vi "多帧发送机制(EV05).vi"(0 "can卡类型":u8, 1 "设备索引号":u8, 2 "CAN端口":u8, 3 "命令":u8 format="%x", 4 "板号":u8 format="%x", 5 "命令序号":u32, 6 "输入数据":dbl[](array[numeric]), 7 "错误输入（无错误）":errorcluster) -> (14 "错误代码":u32, 15 "总发送帧数":i32, 19 "错误输出":errorcluster)   [LabVIEW 2013]
uses:
  data/kerneldlls/usbcan.dll
panel:
  out "发送成功":bool
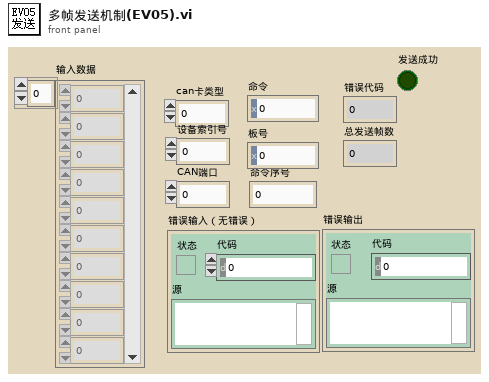
[diagram p1: front panel]
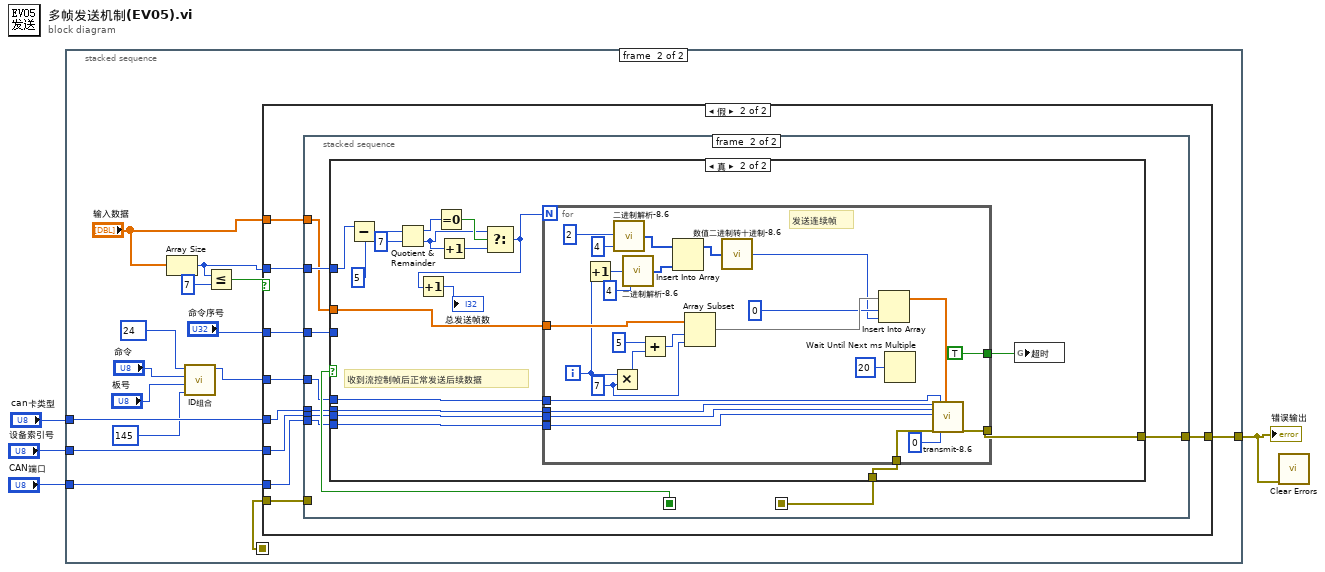
[diagram p0: block diagram]
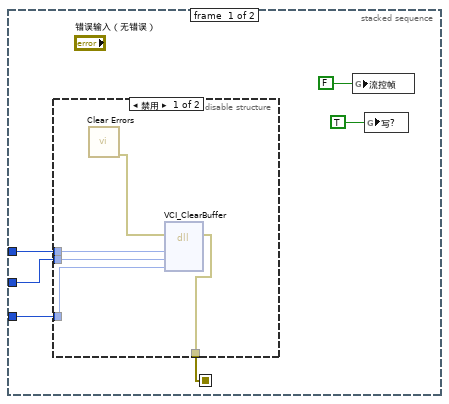
[diagram p2: hidden frame]
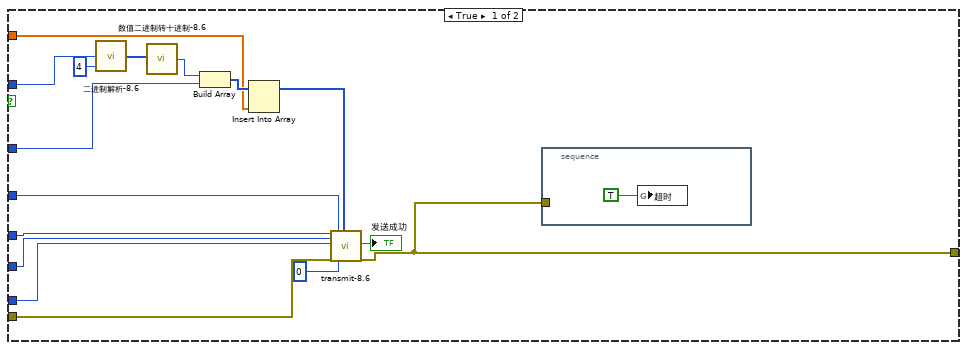
[diagram p4: hidden frame]
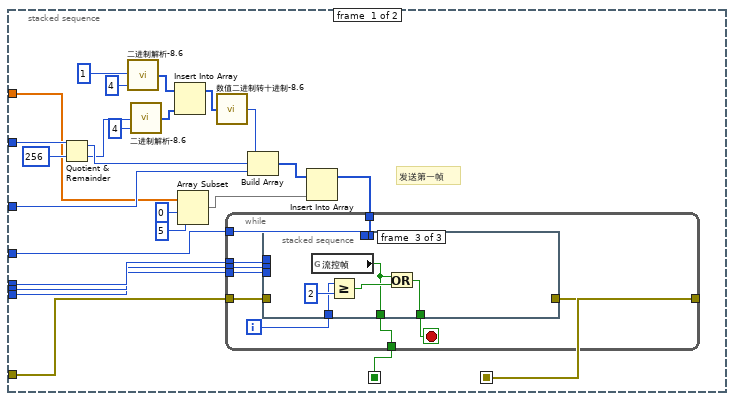
[diagram p5: hidden frame]
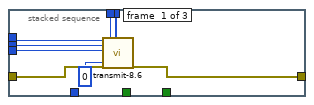
[diagram p6: hidden frame]
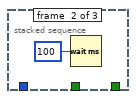
[diagram p7: hidden frame]
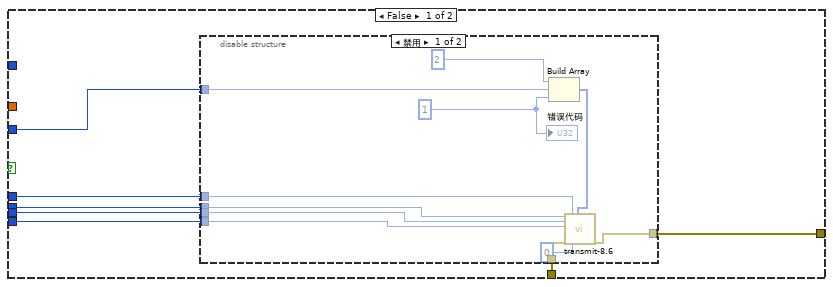
[diagram p8: hidden frame]
diagram:
  n1 = stacked-sequence {
    seq-local: [w7 _] -> [_ w22]
    tunnel: "can卡类型" -> [w10 w25]
    tunnel: "设备索引号" -> [w9 w24]
    tunnel: "CAN端口" -> [w8 w23]
    tunnel: [_ w21] -> w1
    frame #0 {
      n2 = disable-structure shown="禁用" {
        disable-tunnel: w10 -> [w15 _]
        disable-tunnel: w9 -> [w14 _]
        disable-tunnel: w8 -> [w13 _]
        disable-tunnel: [w12 _] -> w7
        frame Disabled {
          n3 = call <vilib>:"Clear Errors.vi"() -> ("error out"=w11:errorcluster)  [unwired: 1 in, 6 out]
          n4 = dll-call lib="PTH1|abs FBluewave New EnergySVN_WorkBMS_Monitor_Bnet01trunkBMS_Monitor_增加二维码data\nkerneldlls\nusbcan.dll" fn="VCI_ClearBuffer"(error in=w11, "DeviceType"=w15, "DeviceInd"=w14, "CANInd"=w13) -> (error out=w12:errorcluster)  [unwired: 2 in, 5 out]
        }
        frame Enabled {
        }
      }
      n5 = global write "EV05全局变量1.vi" "流控帧"(FALSE ("流控帧")) -> ()
      n6 = global write "EV05全局变量1.vi" "写?"(TRUE ("写?")) -> ()
    }
    frame #1 {
      n7 = Array Size(array="输入数据") -> (size(s)=w28:i32)
      n8 = call "ID组合.vi"("SA(4)"=145 ("PDU(1)"), "PS(3)"="板号", "PF(2)"="命令", "PDU(1)"=24) -> ("ID"=w16:i32)  [unwired: 7 out]
      n9 = Less Or Equal?(x=w28, y=7) -> (x <= y?=w29:bool)
      n10 = case shown="假" w29 {
        tunnel: w25 -> [w46 w56]
        tunnel: w24 -> [w45 w55]
        tunnel: w23 -> [w44 w54]
        tunnel: w28 -> [w42 w51]
        tunnel: "命令序号" -> [w43 w53]
        tunnel: "输入数据" -> [w37 w50]
        tunnel: w16 -> [w33 w52]
        tunnel: w22 -> [w35 w49]
        tunnel: [w34 w48] -> w21
        frame True {
          n11 = call "二进制解析-8.6.vi"("索引"=4, "数值"=w42) -> ("低位子数组"=w40:i32[])  [unwired: 3 out]
          n12 = call "数值二进制转十进制-8.6.vi"("子数组"=w40) -> ("十进制数值"=w39:i32)  [unwired: 4 out]
          n13 = Build Array(w39, w43) -> (w38:u32[])
          n14 = Insert Into Array(array=w38, new element=w37) -> (w36:u32[])  [unwired: 1 in]
          n15 = call "transmit-8.6.vi"("can卡类型"=w46, "设备索引号"=w45, "CAN端口"=w44, "错误输入（无错误）"=w35, "ID"=w33, "SendType"=u8 0, "Data"=w36) -> ("发送成功"=→"发送成功":bool, "错误输出"=w34:errorcluster)  [unwired: 2 in, 9 out]
          n16 = stacked-sequence {
            tunnel: w34 -> [_]
            frame #0 {
              n17 = global write "EV05全局变量1.vi" "超时"(TRUE ("超时")) -> ()
            }
          }
        }
        frame False {
          n18 = stacked-sequence {
            seq-local: [w57 _] -> [_ w115]
            seq-local: [w59 _] -> [_ w108]
            tunnel: w56 -> [w81 w111]
            tunnel: w55 -> [w80 w110]
            tunnel: w54 -> [w79 w109]
            tunnel: w53 -> [w78 w106]
            tunnel: w52 -> [w75 w112]
            tunnel: w51 -> [w74 w114]
            tunnel: w50 -> [w64 w113]
            tunnel: w49 -> [w60 _]
            tunnel: [_ w107] -> w48
            frame #0 {
              # "发送第一帧"
              n19 = Quotient & Remainder(x=w74, y=256) -> (x-y*floor(x/y)=w72:i32, floor(x/y)=w71:i32)
              n20 = call "二进制解析-8.6.vi"("索引"=4, "数值"=1) -> ("低位子数组"=w58:i32[])  [unwired: 3 out]
              n21 = call "二进制解析-8.6.vi"("索引"=4, "数值"=w71) -> ("低位子数组"=w67:i32[])  [unwired: 3 out]
              n22 = Insert Into Array(array=w58, new element=w67) -> (w66:i32[])  [unwired: 1 in]
              n23 = Array Subset(array=w64, index=0 ("索引"), length=5 ("长度")) -> (w61:dbl[])
              n24 = call "数值二进制转十进制-8.6.vi"("子数组"=w66) -> ("十进制数值"=w65:i32)  [unwired: 4 out]
              n25 = Build Array(w65, w72, w78) -> (w77:u32[])
              n26 = Insert Into Array(array=w77, new element=w61) -> (w76:u32[])  [unwired: 1 in]
              n27 = while {
                tunnel: w81 -> [w91]
                tunnel: w80 -> [w90]
                tunnel: w79 -> [w89]
                tunnel: w76 -> [w88]
                tunnel: w75 -> [w87]
                tunnel: [w82] -> w57
                tunnel: w60 -> [w86]
                tunnel: [w85] -> w59
                i -> [w84]
                stop <- w83 stop-if-true
                n28 = stacked-sequence {
                  tunnel: w91 -> [w99 _ _]
                  tunnel: w90 -> [w98 _ _]
                  tunnel: w89 -> [w97 _ _]
                  tunnel: w88 -> [w96 _ _]
                  tunnel: w87 -> [w95 _ _]
                  tunnel: w86 -> [w94 _ _]
                  tunnel: [w93 _ _] -> w85
                  tunnel: w84 -> [_ _ w104]
                  tunnel: [_ _ w102] -> w83
                  tunnel: [_ _ w101] -> w82
                  frame #0 {
                    n29 = call "transmit-8.6.vi"("can卡类型"=w99, "设备索引号"=w98, "CAN端口"=w97, "错误输入（无错误）"=w94, "ID"=w95, "SendType"=u8 0, "Data"=w96) -> ("错误输出"=w93:errorcluster)  [unwired: 2 in, 10 out]
                  }
                  frame #1 {
                    n30 = Wait (ms)(milliseconds to wait=u32 100 ("等待时间（毫秒）")) -> ()  [unwired: 1 out]
                  }
                  frame #2 {
                    n31 = global read "EV05全局变量1.vi" "流控帧"() -> (w101:bool)
                    n32 = Greater Or Equal?(x=w104, y=2) -> (x >= y?=w103:bool)
                    n33 = Or(x=w101, y=w103) -> (x .or. y?=w102:bool)
                  }
                }
              }
            }
            frame #1 {
              n34 = case shown="真" w115 {
                tunnel: w114 -> [_ w151]
                tunnel: w113 -> [_ w143]
                tunnel: w112 -> [w116 w142]
                tunnel: w111 -> [w120 w141]
                tunnel: w110 -> [w119 w140]
                tunnel: w109 -> [w118 w139]
                tunnel: w108 -> [w122 w138]
                tunnel: [w121 w137] -> w107
                tunnel: w106 -> [w117 _]
                frame False {
                  n35 = disable-structure shown="禁用" {
                    disable-tunnel: w122 -> [w133 _]
                    disable-tunnel: [w132 _] -> w121
                    disable-tunnel: w120 -> [w131 _]
                    disable-tunnel: w119 -> [w130 _]
                    disable-tunnel: w118 -> [w129 _]
                    disable-tunnel: w117 -> [w126 _]
                    disable-tunnel: w116 -> [w124 _]
                    frame Disabled {
                      w125 = u32 1 ("元素")
                      n36 = Build Array(u8 2 ("元素"), w126, w125) -> (w127:u32[])
                      n37 = call "transmit-8.6.vi"("can卡类型"=w131, "设备索引号"=w130, "CAN端口"=w129, "错误输入（无错误）"=w133, "ID"=w124, "SendType"=u8 0, "Data"=w127) -> ("错误输出"=w132:errorcluster)  [unwired: 2 in, 10 out]
                      "错误代码" <- w125
                    }
                    frame Enabled {
                    }
                  }
                }
                frame True {
                  # "收到流控制帧后正常发送后续数据"
                  n38 = Subtract(x=w151, y=5) -> (x-y=w149:i32)
                  n39 = Quotient & Remainder(x=w149, y=7) -> (x-y*floor(x/y)=w147:i32, floor(x/y)=w145:i32)
                  n40 = Equal To 0?(x=w147) -> (x = 0?=w146:bool)
                  n41 = Increment(x=w145) -> (x+1=w144:i32)
                  n42 = Select(t=w145, s=w146, f=w144) -> (s? t:f=w136:i32)
                  n43 = Increment(x=w136) -> (x+1=→"总发送帧数":i32)
                  n44 = for {
                    N: w136 -> [_]
                    tunnel: w143 -> [w174]
                    tunnel: w142 -> [w163]
                    tunnel: w141 -> [w162]
                    tunnel: w140 -> [w161]
                    tunnel: w139 -> [w160]
                    tunnel: w138 -> [w159]
                    tunnel: [w158] -> w137
                    tunnel: [TRUE] -> w134
                    i -> [w172]
                    w169 = 7 ("y")
                    # "发送连续帧"
                    n45 = Increment(x=w172) -> (x+1=w177:i32)
                    n46 = Multiply(x=w172, y=w169) -> (x*y=w171:i32)
                    n47 = call "二进制解析-8.6.vi"("索引"=4, "数值"=2) -> ("低位子数组"=w153:i32[])  [unwired: 3 out]
                    n48 = call "二进制解析-8.6.vi"("索引"=4, "数值"=w177) -> ("低位子数组"=w175:i32[])  [unwired: 3 out]
                    n49 = Add(x=5 ("索引"), y=w171) -> (x+y=w170:i32)
                    n50 = Insert Into Array(array=w153, new element=w175) -> (w168:i32[])  [unwired: 1 in]
                    n51 = Array Subset(array=w174, index=w170, length=w169) -> (w167:dbl[])
                    n52 = call "数值二进制转十进制-8.6.vi"("子数组"=w168) -> ("十进制数值"=w165:i32)  [unwired: 4 out]
                    n53 = Insert Into Array(array=w167, index=0 ("索引"), new element=w165) -> (w164:dbl[])
                    n54 = Wait Until Next ms Multiple(millisecond multiple=u32 20 ("毫秒倍数")) -> ()  [unwired: 1 out]
                    n55 = call "transmit-8.6.vi"("can卡类型"=w162, "设备索引号"=w161, "CAN端口"=w160, "错误输入（无错误）"=w159, "ID"=w163, "SendType"=u8 0, "Data"=w164) -> ("错误输出"=w158:errorcluster)  [unwired: 2 in, 10 out]
                  }
                  n56 = global write "EV05全局变量1.vi" "超时"(w134) -> ()
                }
              }
            }
          }
        }
      }
    }
  }
  "错误输出" <- w1
  n57 = call <vilib>:"Clear Errors.vi"("error in (no error)"=w1) -> ()  [unwired: 7 out]
